vi "Scope Targets.vi"(9 "Specific Targets":refnum<vi>[](array[refnum]), 10 "Launching VI":refnum<vi>, 11 "Search Scope":T1) -> (3 "Scope Targets":refnum<vi>[](array[refnum]))   [LabVIEW 2016, in "Better Search.lvlib" / "BetterSearch.lvclass"]
uses:
  BetterSearch.lvclass
  Data Types/Search Scope.ctl
  Better Search.lvlib
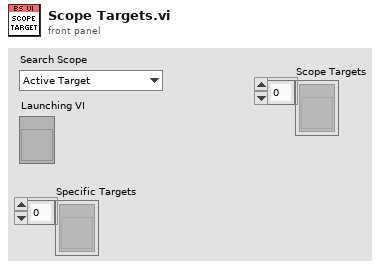
[diagram p1: front panel]
types:
  T1 = typedef "Better Search.lvlib/Search Scope.ctl" = enum16{"Active Target", "Active Project", "Specific Targets", "Active VI", "Active Hierarchy"}
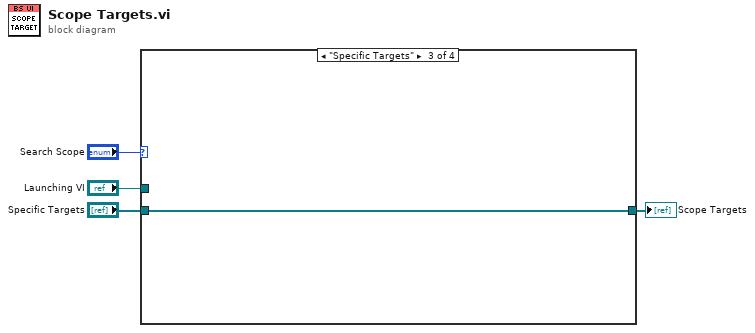
[diagram p0: block diagram]
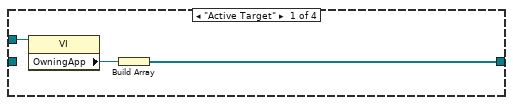
[diagram p2: hidden frame]
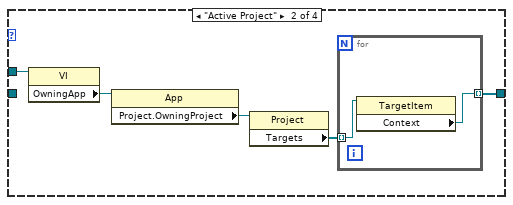
[diagram p3: hidden frame]
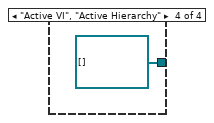
[diagram p4: hidden frame]
diagram:
  n1 = case shown="\"Specific Targets\"" "Search Scope" {
    tunnel: "Launching VI" -> [w7 w12 _ _]
    tunnel: [w5 w8 w15 refnum<vi>[] [] ("Specific Targets")] -> w2
    tunnel: "Specific Targets" -> [_ _ w15 _]
    frame "Active Target" {
      n2 = property class="VI"(reference=w7) -> ("OwningApp"=w6:refnum<vi>)  [unwired: 1 in, 2 out]
      n3 = Build Array(w6) -> (w5:refnum<vi>[])
    }
    frame "Active Project" {
      n4 = property class="VI"(reference=w12) -> ("OwningApp"=w11:refnum<vi>)  [unwired: 1 in, 2 out]
      n5 = property class="App"(reference=w11) -> ("Project.OwningProject"=w10:refnum<vi>)  [unwired: 1 in, 2 out]
      n6 = property class="Project"(reference=w10) -> ("Targets"=w9:refnum<vi>[])  [unwired: 1 in, 2 out]
      n7 = for {
        tunnel: w9 -> [w14] mode=indexing
        tunnel: [w13] -> w8 mode=indexing
        n8 = property class="TargetItem"(reference=w14) -> ("Context"=w13:refnum<vi>)  [unwired: 1 in, 2 out]
      }
    }
    frame "Specific Targets" {
    }
    frame "Active VI", "Active Hierarchy" {
    }
  }
  "Scope Targets" <- w2
